vi "Remove Node.vi"(8 "error in":errorcluster, 11 "Node Guard in":refnum<class "Node Guard.lvclass">) -> (0 "error out":errorcluster, 3 "Node Guard out":refnum<class "Node Guard.lvclass">)   [LabVIEW 2020, in "CANopen.lvlib" / "Network Management.lvlib" / "Node Guard.lvlib" / "Node Guard.lvclass"]
uses:
  Node Guard.lvclass
  Node Guard.lvclass/Node Guard.ctl
  <vilib>/ActorFramework/Time-Delayed Send Message/Time-Delay Override Options.ctl
  <vilib>/ActorFramework/Actor Framework.lvlib
panel:
  in  "Node ID":u8
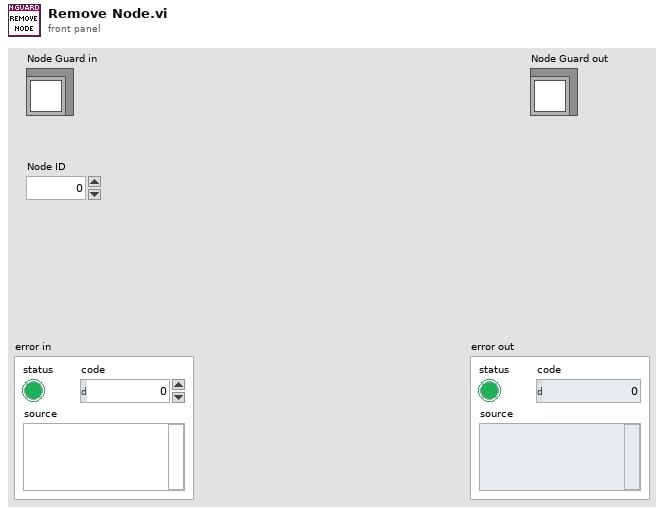
[diagram p1: front panel]
types:
  T1 = typedef "Actor Framework.lvlib/Time-Delay Override Options.ctl" = enum16{"Send next copy now", "Skip next scheduled copy", "Send next copy now and stop all further copies", "Stop all further copies"}
  T2 = map{u8, cluster{"State":u8, "Timings":cluster{"Guard time (ms)":u32, "Lifetime Factor":dbl}, "Toogle Bit":bool, "Delivery Notifier":refnum<notifier>, "Last Received Tick":u32}}
  T3 = cluster{"State":u8, "Timings":cluster{"Guard time (ms)":u32, "Lifetime Factor":dbl}, "Toogle Bit":bool, "Delivery Notifier":refnum<notifier>, "Last Received Tick":u32}
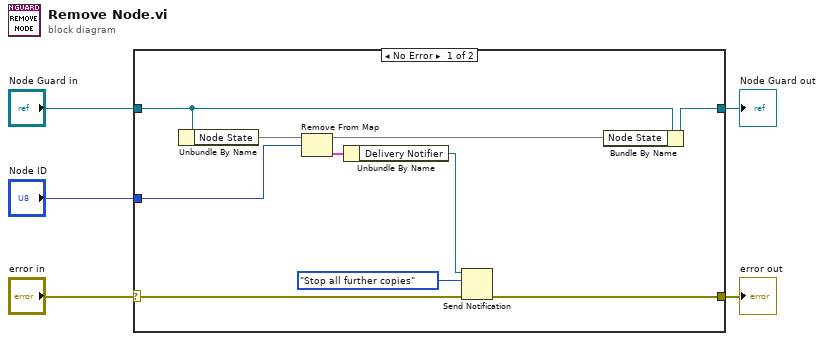
[diagram p0: block diagram]
diagram:
  n1 = case shown="No Error" "error in" {
    selector: "error in" -> [w15 w17]
    tunnel: [w13 w17] -> w2
    tunnel: [w10 w16] -> w4
    tunnel: "Node Guard in" -> [w14 w16]
    tunnel: "Node ID" -> [w7 _]
    frame No Error {
      n2 = Unbundle By Name(w14) -> ("Node State"=w9:T2)
      n3 = Remove From Map(10:w7, 11:w9) -> (1:w6:T3, 3:w8:T2)  [unwired: 1 out]
      n4 = Unbundle By Name(w6) -> ("Delivery Notifier"=w12:refnum<notifier>)
      n5 = Send Notification(notification=Time-Delay_Override_Options."Stop all further copies", notifier=w12, error in (no error)=w15) -> (error out=w13:errorcluster)  [unwired: 1 out]
      n6 = Bundle By Name(cluster=w14, "Node State"=w8) -> (w10:refnum<class "Node Guard.lvclass">)
    }
    frame Error {
    }
  }
  "Node Guard out" <- w4
  "error out" <- w2
